vi "TakeScan.vi"(4 "Target File Path":path=path "C:/Users/Carson/Desktop/Test Scans", 6 "ezAFM Default Path":path=path "D:/ezAFM/Scanned Images", 8 "Angle":dbl, 9 "Image Resolution":u16(ring)=256 items=["32"=32, "64"=64, "128"=128, "256"=256, "512"=512, "1024"=1024, "2048"=2048], 11 "Name":string) -> (2 "Finished?":bool)   [LabVIEW 2015]
panel:
  out "error out":errorcluster
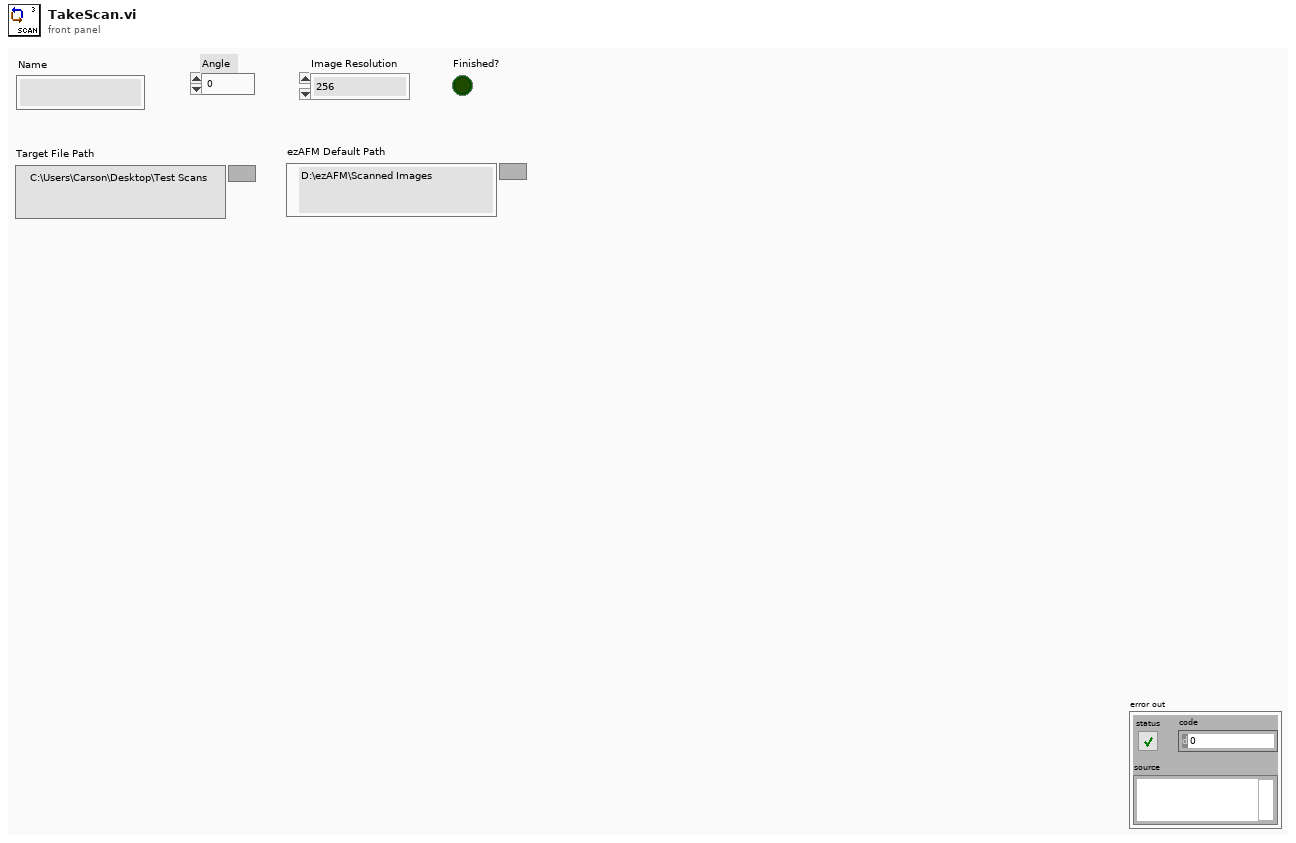
[diagram p1: front panel]
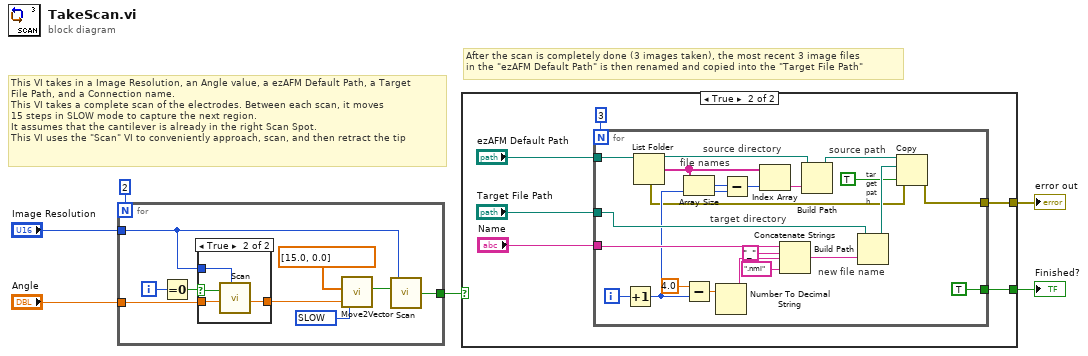
[diagram p0: block diagram]
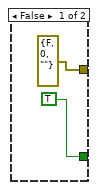
[diagram p2: hidden frame]
diagram:
  # "After the scan is completely done (3 images taken), the most recent 3 image files\nin the \"ezAFM Default Path\" is then renamed and copied into the \"Target File Path\""
  # "This VI takes in a Image Resolution, an Angle value, a ezAFM Default Path, a Target\nFile Path, and a Connection name. \nThis VI takes a complete scan of the electrodes. Between each scan, it moves\n15 steps in SLOW mode to capture the next region.\nIt assumes that the cantilever is already in the right Scan Spot.\nThis VI uses the \"Scan\" VI to conveniently approach, scan, and then retract the tip"
  n1 = for {
    N: 2 -> [_]
    tunnel: [w12] -> w5
    tunnel: "Image Resolution" -> [w8]
    tunnel: "Angle" -> [w7]
    i -> [w11]
    w13 = u16 3300 items=["SLOW"=3300, "MEDIUM"=30000, "FAST"=65000] ("Motor Speed")
    n2 = Equal To 0?(x=w11) -> (x = 0?=w10:bool)
    n3 = case shown="True" w10 {
      selector: w10 -> [_ w17]
      tunnel: w8 -> [_ w19]
      tunnel: [w16 w18] -> w9
      tunnel: w7 -> [w16 w18]
      frame False {
      }
      frame True {
        n4 = call "Scan.vi"("Image Resolution"=w19, "Scanning"=w17) -> ()  [unwired: 1 out]
      }
    }
    n5 = call "Move2Vector.vi"("Motor Speed"=w13, "Angle"=w9, "XY Vector"=dbl[] [15.0, 0.0]) -> ("Finished?"=w14:bool)  [unwired: 8 in]
    n6 = call "Scan.vi"("Image Resolution"=w8, "Scanning"=w14) -> ("Finished?"=w12:bool)
  }
  n7 = case shown="True" w5 {
    tunnel: [TRUE w22] -> w2
    tunnel: [errorcluster {"status"=FALSE, "code"=0, "source"=""} ("error out") w26] -> w1
    frame False {
    }
    frame True {
      n8 = for {
        N: 3 -> [_]
        tunnel: "ezAFM Default Path" -> [w45]
        tunnel: "Target File Path" -> [w44]
        tunnel: "Name" -> [w41]
        tunnel: [w31] -> w26
        tunnel: [TRUE] -> w22
        i -> [w43]
        # "new file name"
        # "target directory"
        # "source directory"
        # "target path"
        # "source path"
        # "file names"
        n9 = Increment(x=w43) -> (x+1=w33:i32)
        n10 = List Folder(path=w45) -> (path out=w28:path, filenames=w32:string[], error out=w30:errorcluster)  [unwired: 3 in, 1 out]
        n11 = Array Size(array=w32) -> (size(s)=w38:i32)
        n12 = Subtract(x=4.0, y=w33) -> (x-y=w34:dbl)
        n13 = Number To Decimal String(number=w34) -> (decimal integer string=w39:string)  [unwired: 1 in]
        n14 = Subtract(x=w38, y=w33) -> (x-y=w37:i32)
        n15 = Index Array(array=w32, index=w37) -> (element=w49:string)
        n16 = Concatenate Strings(w41, "_" ("string"), w39, ".nmi" ("string")) -> (w40:string)
        n17 = Build Path(base path=w28, name or relative path=w49) -> (appended path=w48:path)
        n18 = Build Path(base path=w44, name or relative path=w40) -> (appended path=w47:path)
        n19 = Copy(8:w30, 9:TRUE ("overwrite (F)"), 10:w47, 11:w48) -> (0:w31:errorcluster)  [unwired: 1 in, 2 out]
      }
    }
  }
  "Finished?" <- w2
  "error out" <- w1
